vi "Home MotionSystem.vi"(8 "error in (no error)":errorcluster, 11 "Configuration in":refnum<class "Configuration.lvclass">) -> (0 "error out":errorcluster, 3 "Configuration out":refnum<class "Configuration.lvclass">)   [LabVIEW 2016, in "MotionSystem.lvlib" / "MotionSystem Configuration.lvclass"]
uses:
  <userlib>/Common Components/Hardware/Abstract System/MotionSystem/MotionSystem Config/MotionSystem Configuration.lvclass
  <userlib>/Configuration Dialog Actor/Configuration.lvclass
  <userlib>/Common Components/Hardware/Abstract System/MotionSystem/MotionSystem Config/Home Move Params.ctl
  <userlib>/Common Components/Hardware/Motor/Motor/Home Params.ctl
  <userlib>/Common Components/Hardware/Motor/Motor/Home Mode.ctl
  <userlib>/Common Components/Hardware/Motor/Motor/Home Dir.ctl
  C:/Program Files (x86)/National Instruments/LabVIEW 2016/user.lib/Configuration Dialog Actor/Configuration.lvclass
  C:/Program Files (x86)/National Instruments/LabVIEW 2016/vi.lib/ActorFramework/Actor/Actor.lvclass
  <userlib>/Common Components/Hardware/Abstract System/MotionSystem/MotionSystem Config/MotionSystem Configuration.lvclass/MotionSystem Configuration.ctl
  <vilib>/ActorFramework/Actor/Actor.lvclass/Actor.ctl
  <userlib>/Common Components/Hardware/Motor/Motor/Motor.lvclass/Motor.ctl
  <userlib>/Common Components/Hardware/Abstract Hardware/Hardware.lvclass/Hardware.ctl
  <vilib>/ActorFramework/Message Enqueuer/Message Enqueuer.lvclass/Message Enqueuer.ctl
  G:/tasks/labview/Fermi Utility Framework/Functions/RPS-3DOF Messages/Single Home Move Msg/Single Home Move Msg.lvclass/Single Home Move Msg.ctl
  <userlib>/Common Components/Hardware/Abstract Hardware/Read Label.vi
  <userlib>/Common Components/Hardware/Abstract System/MotionSystem/MotionSystem Config/Accessors/Read Number of Motions.vi
  <userlib>/Common Components/Hardware/Abstract System/MotionSystem/MotionSystem Config/Accessors/Read Array of Motor Configuration Objs.vi
  <userlib>/Common Components/Hardware/Abstract System/MotionSystem/MotionSystem Config/Accessors/Write Array of Motor Configuration Objs.vi
  <vilib>/ActorFramework/Message Enqueuer/Enqueue.vi
  <userlib>/Common Components/Hardware/Motor/Motor/Motor.lvclass
  C:/Program Files (x86)/National Instruments/LabVIEW 2016/user.lib/Common Components/Hardware/Abstract Hardware/Hardware.lvclass
  G:/tasks/labview/Fermi Utility Framework/Functions/RPS-3DOF Messages/Stop All Msg/Stop All Msg.lvclass
  C:/Program Files (x86)/National Instruments/LabVIEW 2016/vi.lib/ActorFramework/Message/Message.lvclass
  G:/tasks/labview/Fermi Utility Framework/Functions/RPS-3DOF Messages/Single Home Move Msg/Single Home Move Msg.lvclass
  <userlib>/Common Components/Hardware/Motor/Motor Config/Accessors/Read Motor Obj.vi
  <vilib>/ActorFramework/Message Priority Queue/Priority Enqueue.vi
  <userlib>/Common Components/Hardware/Motor/Motor Config/Motor Configuration.lvclass
  <vilib>/ActorFramework/Actor/Actor.lvclass
panel:
  in  "select all":bool
  out "Array of Home Status":cluster{"home status":bool}[](array[cluster])
  in  "Array of Home Actions":T1[](array[typedef])
  in  "Home Move Button":bool
  in  "Stop Button":bool
  out "Array of Current Pos":cluster{"current pos":dbl}[](array[cluster])
  in  "Revert":bool
  in  "Apply":bool
  # "status"
  # "current pos"
  # "select"
  # "axis"
  # "mode"
  # "direction"
  # "shift with respect to EZ"
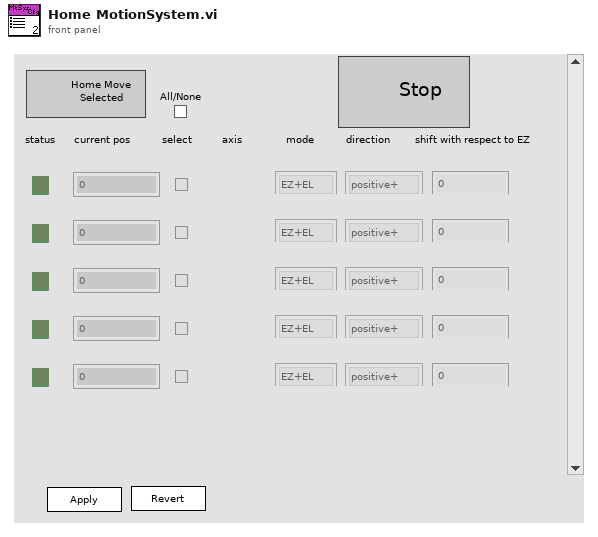
[diagram p1: front panel]
types:
  T1 = typedef "MotionSystem.lvlib/MotionSystem Configuration.lvclass/Home Move Params.ctl" = cluster{"checked?":bool, "label":string, "Home Params Cluster":T2}
  T2 = typedef "Hardware.lvlib/Motor.lvlib/Motor.lvclass/Home Params.ctl" = cluster{"Home Mode":T3, "Home Dir":T4, "Home Pos Shift":dbl}
  T3 = typedef "Hardware.lvlib/Motor.lvlib/Motor.lvclass/Home Mode.ctl" = enum16{"EZ+EL", "EZ only"}
  T4 = typedef "Hardware.lvlib/Motor.lvlib/Motor.lvclass/Home Dir.ctl" = enum16{"negative-", "positive+"}
  T5 = typedef "MotionSystem.lvlib/MotionSystem Configuration.lvclass/Array of Current Pos.ctl" = dbl[]
  T6 = typedef "MotionSystem.lvlib/MotionSystem Configuration.lvclass/Array of Homing Status.ctl" = bool[]
  T7 = cluster{"checked?":bool, "label":bool, "Home Params Cluster":cluster{"Home Mode":bool, "Home Dir":bool, "Home Pos Shift":bool}}[]
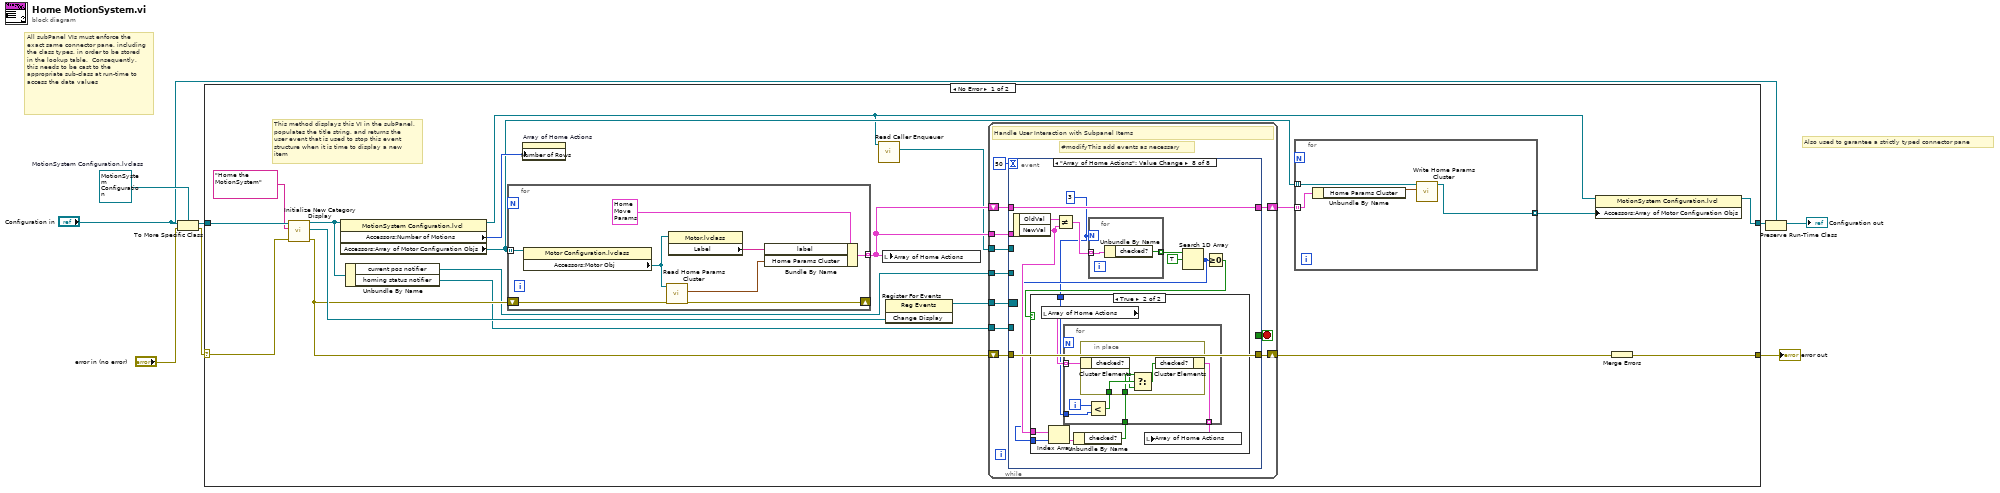
[diagram p0: block diagram]
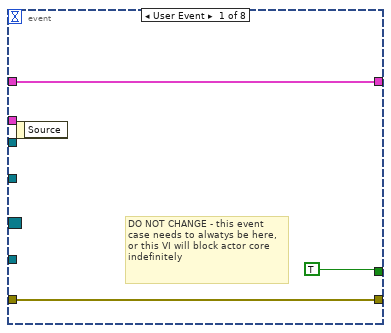
[diagram p2: hidden frame]
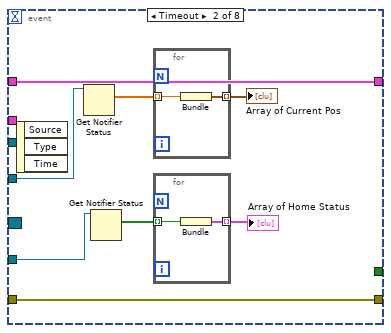
[diagram p3: hidden frame]
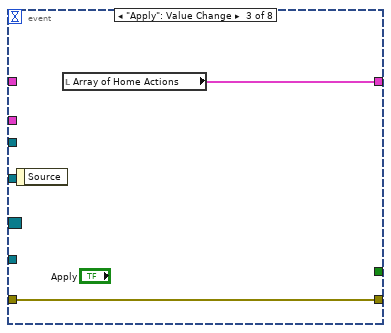
[diagram p4: hidden frame]
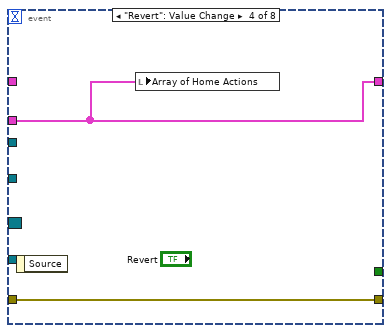
[diagram p5: hidden frame]
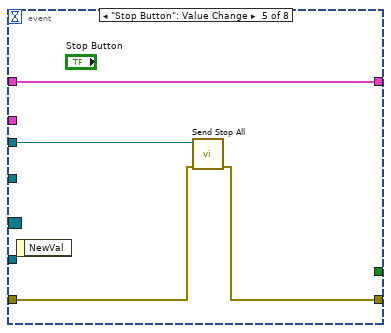
[diagram p6: hidden frame]
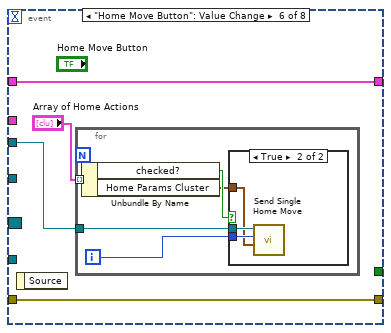
[diagram p7: hidden frame]
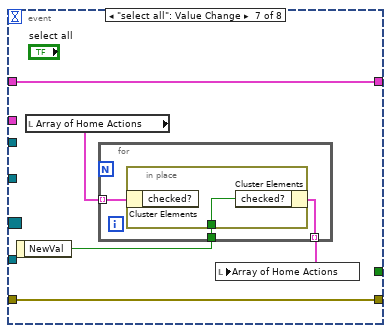
[diagram p9: hidden frame]
diagram:
  w5 = refnum<class "MotionSystem Configuration.lvclass"> refnum  # MotionSystem Configuration.lvclass
  # "Also used to garantee a strictly typed connector pane"
  # "All subPanel VIs must enforce the exact same connector pane, including the class types, in order to be stored in the lookup table.  Consequently, this needs to be cast to the appropriate sub-class at run-time to access the data values"
  n1 = To More Specific Class(target class=w5, reference="Configuration in", error in="error in (no error)") -> (specific class reference=w6:refnum<class "MotionSystem Configuration.lvclass">, error out=w1:errorcluster)
  n2 = case shown="No Error" w1 {
    selector: w1 -> [w13 w124]
    tunnel: w6 -> [w27 w125]
    tunnel: [w21 w125] -> w8
    tunnel: [w26 w124] -> w7
    frame No Error {
      # "This method displays this VI in the subPanel, populates the title string, and returns the user event that is used to stop this event structure when it is time to display a new item"
      n3 = call <userlib>:"Initialize New Category Display.vi"("error in (no error)"=w13, "Name to Display"="Home the MotionSystem", "Configuration in"=w27) -> ("error out"=w14:errorcluster, "Change Display"=w24:refnum<user-event>, "Configuration Out"=w11:refnum<class "MotionSystem Configuration.lvclass">)  [unwired: 6 in]
      n4 = property class="MotionSystem Configuration.lvcl"(reference=w11) -> (reference out=w15:refnum<class "MotionSystem Configuration.lvclass">, "Accessors:Number of Motions"=w20:i32, "Accessors:Array of Motor Configuration Objs"=w18:refnum<class "Motor Configuration.lvclass">[])  [unwired: 1 in, 1 out]
      n5 = Unbundle By Name(w11) -> ("current pos notifier"=w10:refnum<notifier>, "homing status notifier"=w9:refnum<notifier>)
      n6 = for {
        tunnel: w18 -> [w39] mode=indexing
        tunnel: [w37] -> w19 mode=indexing
        shift-right: [w32] -> _
        shift-left: w14 -> [w33]
        n7 = property class="Motor Configuration.lvclass"(reference=w39) -> ("Accessors:Motor Obj"=w35:refnum<class "Motor.lvclass">)  [unwired: 1 in, 2 out]
        n8 = call <userlib>:"Read Home Params Cluster.vi"("error in (no error)"=w33, "Motor in"=w35) -> ("error out"=w32:errorcluster, "Home Params Cluster"=w34:T2)  [unwired: 7 in, 1 out]
        n9 = property class="Motor.lvclass"(reference=w35) -> ("Label"=w36:string)  [unwired: 1 in, 2 out]
        n10 = Bundle By Name(cluster=T1 {"checked?"=FALSE, "label"="", "Home Params Cluster"={"Home Mode"=enum."EZ+EL", "Home Dir"=enum."positive+", "Home Pos Shift"=0.0}} ("Cluster"), "label"=w36, "Home Params Cluster"=w34) -> (w37:T1)
      }
      n11 = property on="Array of Home Actions" class="Arr (strict)"("Number of Rows"=w20) -> ()  [unwired: 2 in, 2 out]
      n12 = call <vilib>:"Read Caller Enqueuer.vi"("Actor"=w15) -> ("Caller Enqueuer"=w12:refnum<class "Message Enqueuer.lvclass">)  [unwired: 10 in]
      n13 = local write "Array of Home Actions"(w19) -> ()
      n14 = register-events(w24) -> (reference out=w23:refnum<event-registration>)  [unwired: 2 in, 1 out]
      n15 = while {
        tunnel: w23 -> [w49]
        shift-right: [w48] -> w22
        shift-left: w14 -> [w47]
        shift-right: [w45] -> w17
        shift-left: w19 -> [w46]
        tunnel: w19 -> [w44]
        tunnel: w12 -> [w43]
        tunnel: w10 -> [w41]
        tunnel: w9 -> [w40]
        stop <- w50 stop-if-true
        # "#modifyThis add events as necessary"
        # "Handle User Interaction with Subpanel Items"
        n16 = event shown="[7] \"Array of Home Actions\": Value Change" {
          selector: w49 -> [_ _ _ _ _ _ _ _]
          dyn-events: _ -> [_ _ _ _ _ _ _ _]
          timeout: 50 -> [_ _ _ _ _ _ _ _]
          tunnel: [TRUE _ _ _ _ _ _ _] -> w50
          tunnel: [w53 w61 w67 w69 w70 w77 w90 w104] -> w48
          tunnel: w47 -> [w53 w61 w67 w69 w71 w77 w90 w104]
          tunnel: w46 -> [w52 w60 _ _ w73 w76 w89 w103]
          tunnel: [w52 w60 w66 w68 w73 w76 w89 w103] -> w45
          tunnel: w44 -> [_ _ _ w68 _ _ _ _]
          tunnel: w43 -> [_ _ _ _ w72 w74 _ _]
          tunnel: w41 -> [_ w59 _ _ _ _ _ _]
          tunnel: w40 -> [_ w58 _ _ _ _ _ _]
          event User Event {
            # "DO NOT CHANGE - this event case needs to alwatys be here, or this VI will block actor core indefinitely"
            n17 = event-data() -> ()  [unwired: 1 in, 1 out]
          }
          event Timeout {
            n18 = event-data() -> ()  [unwired: 1 in, 3 out]
            n19 = Get Notifier Status(notifier=w59) -> (current notification=w55:T5)  [unwired: 1 in, 4 out]
            n20 = Get Notifier Status(notifier=w58) -> (current notification=w54:T6)  [unwired: 1 in, 4 out]
            n21 = for {
              tunnel: w55 -> [w65] mode=indexing
              tunnel: [w64] -> w56 mode=indexing
              n22 = Bundle("encoder pos in unit mode"=w65) -> (w64:cluster{"encoder pos in unit mode":dbl})  [unwired: 1 in]
            }
            "Array of Current Pos" <- w56
            n23 = for {
              tunnel: w54 -> [w63] mode=indexing
              tunnel: [w62] -> w57 mode=indexing
              n24 = Bundle("Boolean"=w63) -> (w62:cluster{"Boolean":bool})  [unwired: 1 in]
            }
            "Array of Home Status" <- w57
          }
          event "Apply": Value Change {
            n25 = event-data() -> ()  [unwired: 1 in, 1 out]
            n26 = local read "Array of Home Actions"() -> (w66:T1[])
          }
          event "Revert": Value Change {
            n27 = event-data() -> ()  [unwired: 1 in, 1 out]
            n28 = local write "Array of Home Actions"(w68) -> ()
          }
          event "Stop Button": Value Change {
            n29 = event-data() -> ()  [unwired: 1 in, 1 out]
            n30 = call "Send Stop All.vi"("error in (no error)"=w71, "Message Enqueuer"=w72) -> ("error out"=w70:errorcluster)  [unwired: 8 in, 1 out]
          }
          event "Home Move Button": Value Change {
            n31 = event-data() -> ()  [unwired: 1 in, 1 out]
            n32 = for {
              tunnel: "Array of Home Actions" -> [w82] mode=indexing
              tunnel: w74 -> [w80]
              i -> [w79]
              n33 = Unbundle By Name(w82) -> ("checked?"=w81:bool, "Home Params Cluster"=w78:T2)
              n34 = case shown="True" w81 {
                tunnel: w80 -> [_ w85]
                tunnel: w79 -> [_ w84]
                tunnel: w78 -> [_ w83]
                frame False {
                }
                frame True {
                  n35 = call "Send Single Home Move.vi"("Home Params Cluster"=w83, "index (0-based)"=w84, "Message Enqueuer"=w85) -> ()  [unwired: 7 in, 2 out]
                }
              }
            }
          }
          event "select all": Value Change {
            n36 = event-data() -> ("NewVal"=w87:bool)  [unwired: 1 in]
            n37 = local read "Array of Home Actions"() -> (w88:T1[])
            n38 = for {
              tunnel: w88 -> [w93] mode=indexing
              tunnel: w87 -> [w92]
              tunnel: [w91] -> w86 mode=indexing
              n39 = in-place {
                in-place-border: w92 -> [w94]
                n40 = in-place-cluster #1(w93) -> ()  [unwired: 1 out]
                n41 = in-place-cluster #1("checked?"=w94) -> (w91:T1)
              }
            }
            n42 = local write "Array of Home Actions"(w86) -> ()
          }
          event "Array of Home Actions": Value Change {
            w95 = 3
            n43 = event-data() -> ("OldVal"=w102:T1[], "NewVal"=w97:T1[])  [unwired: 1 in]
            n44 = Not Equal?(x=w102, y=w97) -> (x != y?=w101:T7)
            n45 = for {
              N: w95 -> [_]
              tunnel: w101 -> [w123] mode=indexing
              tunnel: [w122] -> w100 mode=indexing
              n46 = Unbundle By Name(w123) -> ("checked?"=w122:bool)
            }
            n47 = Search 1D Array(1D array=w100, element=TRUE) -> (index of element=w96:i32)  [unwired: 1 in]
            n48 = Greater Or Equal To 0?(x=w96) -> (x >= 0?=w98:bool)
            n49 = case shown="True" w98 {
              tunnel: w97 -> [_ w109]
              tunnel: w96 -> [_ w108]
              tunnel: w95 -> [_ w106]
              frame False {
              }
              frame True {
                n50 = local read "Array of Home Actions"() -> (w110:T1[])
                n51 = Index Array(array=w109, index=w108) -> (element=w107:T1)
                n52 = Unbundle By Name(w107) -> ("checked?"=w105:bool)
                n53 = for {
                  tunnel: w110 -> [w117] mode=indexing
                  tunnel: [w116] -> w111 mode=indexing
                  tunnel: w106 -> [w114]
                  tunnel: w105 -> [w112]
                  i -> [w115]
                  n54 = Less?(x=w115, y=w114) -> (x < y?=w113:bool)
                  n55 = in-place {
                    in-place-border: w113 -> [w121]
                    in-place-border: w112 -> [w119]
                    n56 = in-place-cluster #2(w117) -> ("checked?"=w118:bool)
                    n57 = Select(t=w119, s=w121, f=w118) -> (s? t:f=w120:bool)
                    n58 = in-place-cluster #2("checked?"=w120) -> (w116:T1)
                  }
                }
                n59 = local write "Array of Home Actions"(w111) -> ()
              }
            }
          }
        }
      }
      n60 = for {
        tunnel: w18 -> [w31] mode=indexing
        tunnel: w17 -> [w30] mode=indexing
        tunnel: [w28] -> w16 mode=indexing
        n61 = Unbundle By Name(w30) -> ("Home Params Cluster"=w29:T2)
        n62 = call <userlib>:"Write Home Params Cluster.vi"("Home Params Cluster"=w29, "Motor Configuration in"=w31) -> ("Motor Configuration out"=w28:refnum<class "Motor Configuration.lvclass">)  [unwired: 8 in, 1 out]
      }
      n63 = property class="MotionSystem Configuration.lvcl"(reference=w15, "Accessors:Array of Motor Configuration Objs"=w16) -> (reference out=w21:refnum<class "MotionSystem Configuration.lvclass">)  [unwired: 1 in, 1 out]
      n64 = Merge Errors(w22) -> (w26:errorcluster)
    }
    frame Error {
    }
  }
  "error out" <- w7
  n65 = Preserve Run-Time Class(object in=w8, 2:"Configuration in") -> (object out=→"Configuration out":refnum<class "Configuration.lvclass">)  [unwired: 1 in, 1 out]
